vi "Autonomous.vi"   [LabVIEW 2015]
doc: "This VI starts when autonomous period begins, and will automatically be terminated when it ends. You can carry out timed or sensor driven operations directly to I/O or to subsystems without needing to return to the caller."
uses:
  <vilib>/Rock Robotics/Network Tables/NT Read String.vi
  <vilib>/Rock Robotics/Network Tables/NT Read Number.vi
  Framework/Robot Global Data.vi
  AutoTask/Implementation/AutoTask Operations.ctl
  AutoTask/Implementation/AutoTask Setpoints.ctl
  NavX/navX Library v2/navX Library v2.lvlib
types:
  T1 = typedef "AutoTask Setpoints.ctl" = cluster{"Operation":T2, "Setpoint":dbl, "Duration":dbl, "Speed":dbl, "Angle":dbl, "VDeadband":dbl, "Deadband":dbl}
  T2 = typedef "AutoTask Operations.ctl" = enum16{"Reserve", "Read Current", "Immediate", "DriveDistance", "AutoShoot", "FaceForward", "AutoAlign", "AutoTurn", "DriveToLine", "DriveToIncline", "DriveTillFlat"}
  T3 = typedef "navX Library v2.lvlib/Z900_navX_DeviceTypeDef.ctl" = cluster{"Interface":cluster{"Protocol":T4, "Update Rate (4Hz-60Hz)":u8, "navX Open TypeDef":variant}, "Notify Packet":refnum<notifier>, "Loop VI Refnum":refnum<vi>, "Ready to Close Occurrence Refnum":refnum<k4>}
  T4 = typedef "navX Library v2.lvlib/Z900_navX_ProtocolTypeDef.ctl" = enum16{"SERIAL", "I2C", "SPI"}
  T5 = cluster{"Yaw":dbl, "Roll":dbl, "Pitch":dbl, "Heading":dbl, "Fused Heading":dbl}
  T6 = typedef "WPI_EncoderDevRef.ctl" = cluster{"DevStatus":errorcluster, "EncoderIndex":T7, "CounterIndex":T8, "DistancePerCount":dbl, "Decoding Type":T9}
  T7 = typedef "FPGA_EncoderIdx.ctl" = enum8{"Enc 0", "Enc 1", "Enc 2", "Enc 3", "Enc 4", "Enc 5", "Enc 6", "Enc 7", "Invalid"}
  T8 = typedef "FPGA_CounterCtrSystemIndex.ctl" = enum8{"Ctr 0", "Ctr 1", "Ctr 2", "Ctr 3", "Ctr 4", "Ctr 5", "Ctr 6", "Ctr 7", "Invalid"}
  T9 = typedef "WPI_EncoderType.ctl" = enum16{"1x", "2x", "4x"}
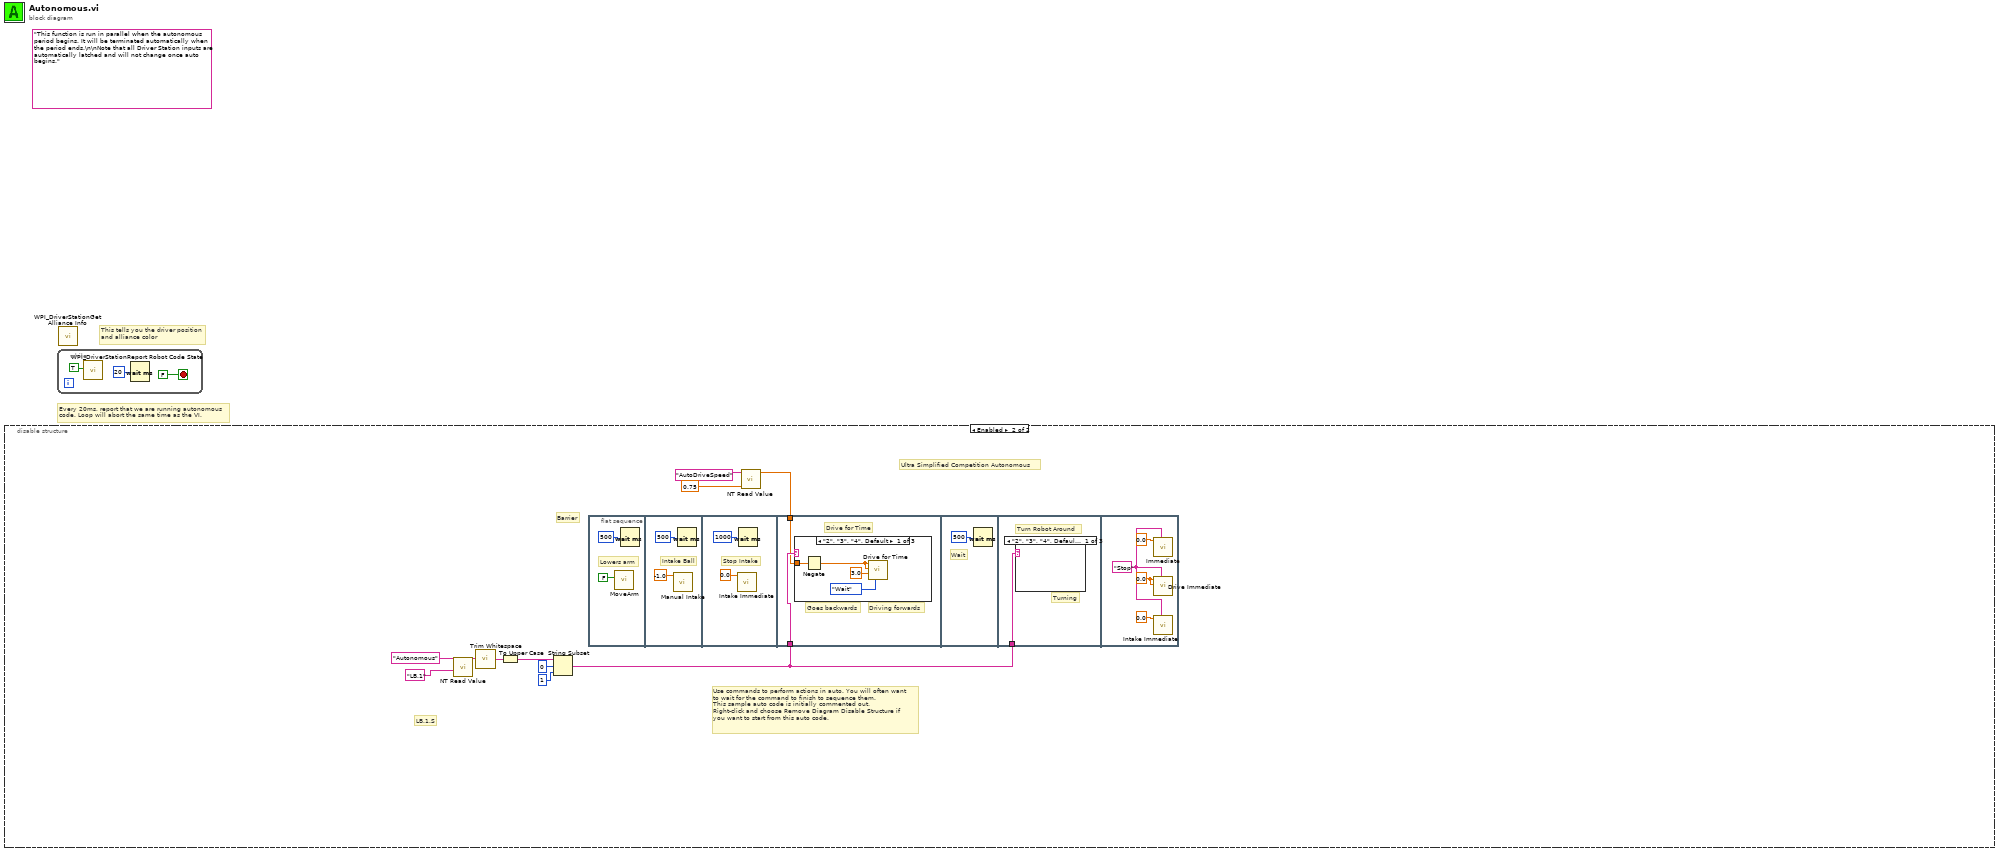
[diagram p0: block diagram]
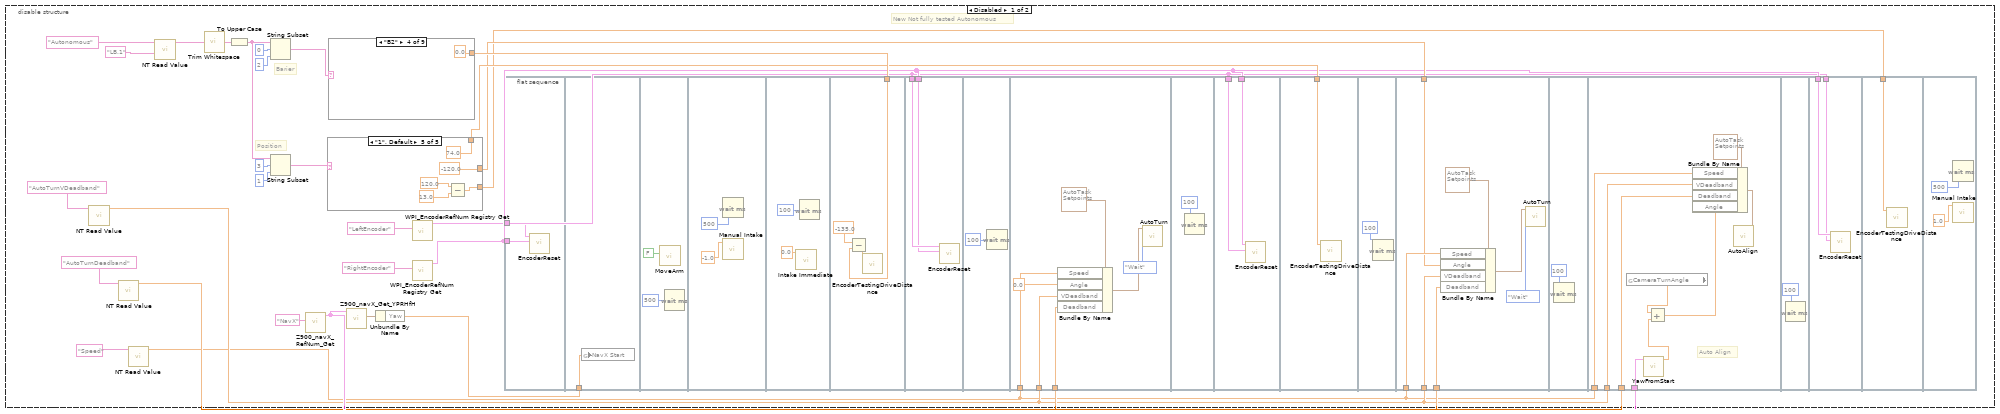
[diagram p2: hidden frame]
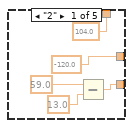
[diagram p3: hidden frame]
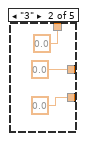
[diagram p4: hidden frame]
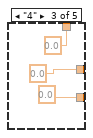
[diagram p5: hidden frame]
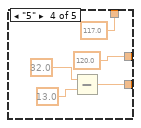
[diagram p6: hidden frame]
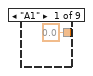
[diagram p7: hidden frame]
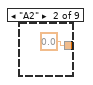
[diagram p8: hidden frame]
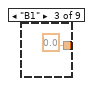
[diagram p9: hidden frame]
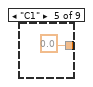
[diagram p10: hidden frame]
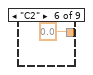
[diagram p11: hidden frame]
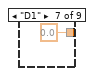
[diagram p12: hidden frame]
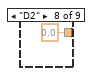
[diagram p13: hidden frame]
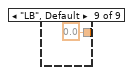
[diagram p14: hidden frame]
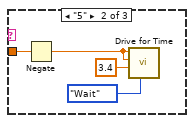
[diagram p15: hidden frame]
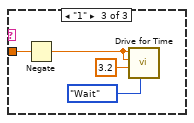
[diagram p16: hidden frame]
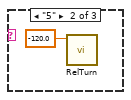
[diagram p17: hidden frame]
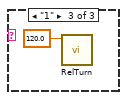
[diagram p18: hidden frame]
diagram:
  (unwired) "This function is run in parallel when the autonomous period begins. It will be terminated automatically when the period ends.\n\nNote that all Driver Station inputs are automatically latched and will not change once auto begins."
  # "Every 20ms, report that we are running autonomous\ncode. Loop will abort the same time as the VI."
  # "This tells you the driver position\nand alliance color"
  n1 = disable-structure shown="Enabled" {
    frame Disabled {
      # "New Not fully tested Autonomous"
      # "Barier"
      # "Position"
      n2 = call-poly <vilib>:"NT Read Value.vi"("Name"="AutoTurnVDeadband") -> ("Numeric"=w5:dbl)  [unwired: 9 in, 1 out]
      n3 = call-poly <vilib>:"NT Read Value.vi"("Name"="AutoTurnDeadband") -> ("Numeric"=w6:dbl)  [unwired: 9 in, 1 out]
      n4 = call-poly <vilib>:"NT Read Value.vi"("Name"="Speed") -> ("Numeric"=w4:dbl)  [unwired: 9 in, 1 out]
      n5 = call-poly <vilib>:"NT Read Value.vi"("Default Value"="LB.1", "Name"="Autonomous") -> ("String"=w23:string)  [unwired: 8 in, 1 out]
      n6 = call <vilib>:"Trim Whitespace.vi"("string"=w23) -> ("trimmed string"=w24:string)  [unwired: 1 in]
      n7 = To Upper Case(1:w24) -> (0:w21:string)
      n8 = String Subset(string=w21, offset (0)=0, length (rest)=2 ("length (rest)")) -> (substring=w20:string)
      n9 = String Subset(string=w21, offset (0)=3, length (rest)=1 ("length (rest)")) -> (substring=w10:string)
      n10 = call "Z900_navX_RefNum_Get.vi"("refnum name"="NavX") -> ("navX Device"=w7:T3)  [unwired: 9 in, 1 out]
      n11 = case shown="\"1\", Default" w10 {
        tunnel: [104.0 ("Distance") 0.0 ("Distance") 0.0 ("Distance") 117.0 ("Distance") 74.0 ("Distance")] -> w9
        tunnel: [-120.0 ("Distance") 0.0 ("Distance") 0.0 ("Distance") 120.0 ("Distance") -120.0 ("Distance")] -> w8
        tunnel: [w30 0.0 ("Distance") 0.0 ("Distance") w43 w48] -> w1
        frame "2" {
          n12 = Subtract(x=59.0 ("Distance"), y=13.0 ("Distance")) -> (x-y=w30:dbl)
        }
        frame "3" {
        }
        frame "4" {
        }
        frame "5" {
          n13 = Subtract(x=32.0 ("Distance"), y=13.0 ("Distance")) -> (x-y=w43:dbl)
        }
        frame "1", Default {
          n14 = Subtract(x=120.0 ("Distance"), y=13.0 ("Distance")) -> (x-y=w48:dbl)
        }
      }
      n15 = case shown="\"B2\"" w20 {
        tunnel: [0.0 ("Distance") 0.0 ("Distance") 0.0 ("Distance") 0.0 ("Distance") 0.0 ("Distance") 0.0 ("Distance") 0.0 ("Distance") 0.0 ("Distance") 0.0 ("Distance")] -> w14
        frame "A1" {
        }
        frame "A2" {
        }
        frame "B1" {
        }
        frame "B2" {
        }
        frame "C1" {
        }
        frame "C2" {
        }
        frame "D1" {
        }
        frame "D2" {
        }
        frame "LB", Default {
        }
      }
      n16 = call "Z900_navX_Get_YPRHfH.vi"("navX Device"=w7) -> ("YRPHfH"=w17:T5)  [unwired: 7 in, 3 out]
      n17 = Unbundle By Name(w17) -> ("Yaw"=w15:dbl)
      n18 = call <vilib>:"WPI_EncoderRefNum Registry Get.vi"("refnum name"="LeftEncoder") -> ("EncoderDevRef"=w2:T6)  [unwired: 9 in, 1 out]
      n19 = call <vilib>:"WPI_EncoderRefNum Registry Get.vi"("refnum name"="RightEncoder") -> ("EncoderDevRef"=w3:T6)  [unwired: 9 in, 1 out]
      n20 = flat-sequence {
        tunnel: w3 -> [w52]
        tunnel: w2 -> [w51]
        tunnel: w15 -> [w53]
        tunnel: w14 -> [w60]
        tunnel: w2 -> [w64]
        tunnel: w3 -> [w63]
        tunnel: w6 -> [w69]
        tunnel: w5 -> [w68]
        tunnel: w4 -> [w67]
        tunnel: w3 -> [w75]
        tunnel: w2 -> [w74]
        tunnel: w9 -> [w76]
        tunnel: w4 -> [w81]
        tunnel: w5 -> [w80]
        tunnel: w6 -> [w79]
        tunnel: w8 -> [w78]
        tunnel: w7 -> [w89]
        tunnel: w6 -> [w88]
        tunnel: w5 -> [w87]
        tunnel: w4 -> [w86]
        tunnel: w3 -> [w97]
        tunnel: w2 -> [w96]
        tunnel: w1 -> [w98]
        frame #0 {
          n21 = call "EncoderReset.vi"("EncoderDevRef 2"=w52, "EncoderDevRef"=w51) -> ()  [unwired: 10 in]
        }
        frame #1 {
          n22 = global write "Robot Global Data.vi" "NavX Start"(w53) -> ()
        }
        frame #2 {
          n23 = call "MoveArm.vi"("OnOff"=FALSE) -> ()  [unwired: 10 in, 1 out]
          n24 = Wait (ms)(milliseconds to wait=u32 500) -> ()  [unwired: 1 out]
        }
        frame #3 {
          n25 = Wait (ms)(milliseconds to wait=u32 500) -> ()  [unwired: 1 out]
          n26 = call "Manual Intake.vi"("Setpoint"=-1.0) -> ()  [unwired: 10 in, 1 out]
        }
        frame #4 {
          n27 = call "Intake Immediate.vi"("Setpoint"=0.0) -> ()  [unwired: 10 in, 1 out]
          n28 = Wait (ms)(milliseconds to wait=u32 100) -> ()  [unwired: 1 out]
        }
        frame #5 {
          n29 = Subtract(x=-135.0 ("Distance"), y=w60) -> (x-y=w61:dbl)
          n30 = call "EncoderTestingDriveDistance.vi"("Distance"=w61) -> ()  [unwired: 11 in]
        }
        frame #6 {
          n31 = call "EncoderReset.vi"("EncoderDevRef 2"=w63, "EncoderDevRef"=w64) -> ()  [unwired: 10 in]
        }
        frame #7 {
          n32 = Wait (ms)(milliseconds to wait=u32 100) -> ()  [unwired: 1 out]
        }
        frame #8 {
          n33 = Bundle By Name(cluster=T1 {"Operation"=enum."Reserve", "Setpoint"=0.0, "Duration"=0.0, "Speed"=0.0, "Angle"=0.0, "VDeadband"=0.0, "Deadband"=0.0} ("SubSystem Data"), "Speed"=w67, "Angle"=0.0, "VDeadband"=w68, "Deadband"=w69) -> (w70:T1)
          n34 = call "AutoTurn.vi"("Synchronization"=enum16{"Start", "Wait"}."Wait", "SubSystem Data"=w70) -> ()  [unwired: 8 in, 1 out]
        }
        frame #9 {
          n35 = Wait (ms)(milliseconds to wait=u32 100) -> ()  [unwired: 1 out]
        }
        frame #10 {
          n36 = call "EncoderReset.vi"("EncoderDevRef 2"=w74, "EncoderDevRef"=w75) -> ()  [unwired: 10 in]
        }
        frame #11 {
          n37 = call "EncoderTestingDriveDistance.vi"("Distance"=w76) -> ()  [unwired: 11 in]
        }
        frame #12 {
          n38 = Wait (ms)(milliseconds to wait=u32 100) -> ()  [unwired: 1 out]
        }
        frame #13 {
          n39 = Bundle By Name(cluster=T1 {"Operation"=enum."Reserve", "Setpoint"=0.0, "Duration"=0.0, "Speed"=0.0, "Angle"=0.0, "VDeadband"=0.0, "Deadband"=0.0} ("SubSystem Data"), "Speed"=w81, "Angle"=w78, "VDeadband"=w80, "Deadband"=w79) -> (w82:T1)
          n40 = call "AutoTurn.vi"("Synchronization"=enum16{"Start", "Wait"}."Wait", "SubSystem Data"=w82) -> ()  [unwired: 8 in, 1 out]
        }
        frame #14 {
          n41 = Wait (ms)(milliseconds to wait=u32 100) -> ()  [unwired: 1 out]
        }
        frame #15 {
          # "Auto Align"
          n42 = global read "Robot Global Data.vi" "CameraTurnAngle"() -> (w92:dbl)
          n43 = call "YawFromStart.vi"("navX Device"=w89) -> ("Yaw"=w93:dbl)  [unwired: 10 in]
          n44 = Add(x=w92, y=w93) -> (x+y=w94:dbl)
          n45 = Bundle By Name(cluster=T1 {"Operation"=enum."AutoAlign", "Setpoint"=0.0, "Duration"=0.0, "Speed"=0.0, "Angle"=0.0, "VDeadband"=0.0, "Deadband"=0.0} ("SubSystem Data"), "Speed"=w86, "VDeadband"=w87, "Deadband"=w88, "Angle"=w94) -> (w90:T1)
          n46 = call "AutoAlign.vi"("SubSystem Data"=w90) -> ()  [unwired: 10 in, 1 out]
        }
        frame #16 {
          n47 = Wait (ms)(milliseconds to wait=u32 100) -> ()  [unwired: 1 out]
        }
        frame #17 {
          n48 = call "EncoderReset.vi"("EncoderDevRef 2"=w96, "EncoderDevRef"=w97) -> ()  [unwired: 10 in]
        }
        frame #18 {
          n49 = call "EncoderTestingDriveDistance.vi"("Distance"=w98) -> ()  [unwired: 11 in]
        }
        frame #19 {
          n50 = Wait (ms)(milliseconds to wait=u32 500) -> ()  [unwired: 1 out]
          n51 = call "Manual Intake.vi"("Setpoint"=1.0) -> ()  [unwired: 10 in, 1 out]
        }
      }
    }
    frame Enabled {
      # "Ultra Simplified Competition Autonomous"
      # "LB.1.S"
      # "Barrier"
      # "Use commands to perform actions in auto. You will often want\nto wait for the command to finish to sequence them.\nThis sample auto code is initially commented out. \nRight-click and choose Remove Diagram Disable Structure if\nyou want to start from this auto code."
      n52 = call-poly <vilib>:"NT Read Value.vi"("Default Value"="LB.1", "Name"="Autonomous") -> ("String"=w112:string)  [unwired: 8 in, 1 out]
      n53 = call <vilib>:"Trim Whitespace.vi"("string"=w112) -> ("trimmed string"=w113:string)  [unwired: 1 in]
      n54 = To Upper Case(1:w113) -> (0:w114:string)
      n55 = String Subset(string=w114, offset (0)=0, length (rest)=1 ("length (rest)")) -> (substring=w116:string)
      n56 = flat-sequence {
        tunnel: w116 -> [w128]
        tunnel: w119 -> [w127]
        tunnel: w116 -> [w142]
        frame #0 {
          # "Lowers arm"
          n57 = call "MoveArm.vi"("OnOff"=FALSE) -> ()  [unwired: 10 in, 1 out]
          n58 = Wait (ms)(milliseconds to wait=u32 500) -> ()  [unwired: 1 out]
        }
        frame #1 {
          # "Intake Ball"
          n59 = call "Manual Intake.vi"("Setpoint"=-1.0) -> ()  [unwired: 10 in, 1 out]
          n60 = Wait (ms)(milliseconds to wait=u32 500) -> ()  [unwired: 1 out]
        }
        frame #2 {
          # "Stop Intake"
          n61 = call "Intake Immediate.vi"("Setpoint"=0.0) -> ()  [unwired: 10 in, 1 out]
          n62 = Wait (ms)(milliseconds to wait=u32 1000) -> ()  [unwired: 1 out]
        }
        frame #3 {
          # "Drive for Time"
          # "Goes backwards"
          # "Driving forwards"
          n63 = case shown="\"2\", \"3\", \"4\", Default" w128 {
            tunnel: w127 -> [w129 w133 w137]
            frame "2", "3", "4", Default {
              n64 = Negate(x=w129) -> (-x=w130:dbl)
              n65 = call "Drive for Time.vi"("Synchronization"=enum16{"Start", "Wait"}."Wait", "Seconds"=3.0, "Right Speed"=w130, "Left Speed"=w130) -> ()  [unwired: 6 in, 2 out]
            }
            frame "5" {
              n66 = Negate(x=w133) -> (-x=w134:dbl)
              n67 = call "Drive for Time.vi"("Synchronization"=enum16{"Start", "Wait"}."Wait", "Seconds"=3.4, "Right Speed"=w134, "Left Speed"=w134) -> ()  [unwired: 6 in, 2 out]
            }
            frame "1" {
              n68 = Negate(x=w137) -> (-x=w138:dbl)
              n69 = call "Drive for Time.vi"("Synchronization"=enum16{"Start", "Wait"}."Wait", "Seconds"=3.2, "Right Speed"=w138, "Left Speed"=w138) -> ()  [unwired: 6 in, 2 out]
            }
          }
        }
        frame #4 {
          # "Wait"
          n70 = Wait (ms)(milliseconds to wait=u32 500) -> ()  [unwired: 1 out]
        }
        frame #5 {
          # "Turn Robot Around"
          # "Turning"
          n71 = case shown="\"2\", \"3\", \"4\", Default" w142 {
            frame "2", "3", "4", Default {
            }
            frame "5" {
              n72 = call "RelTurn.vi"("Angle"=-120.0) -> ()  [unwired: 11 in]
            }
            frame "1" {
              n73 = call "RelTurn.vi"("Angle"=120.0) -> ()  [unwired: 11 in]
            }
          }
        }
        frame #6 {
          w145 = "Stop" ("Description")
          w148 = 0.0
          n74 = call "Immediate.vi"("Description"=w145, "Setpoint"=0.0) -> ()  [unwired: 9 in, 1 out]
          n75 = call "Drive Immediate.vi"("Description"=w145, "Right Setpoint"=w148, "Left Setpoint"=w148) -> ()  [unwired: 8 in, 1 out]
          n76 = call "Intake Immediate.vi"("Description"=w145, "Setpoint"=0.0) -> ()  [unwired: 9 in, 1 out]
        }
      }
      n77 = call-poly <vilib>:"NT Read Value.vi"("Default Value"=0.75, "Name"="AutoDriveSpeed") -> ("Numeric"=w119:dbl)  [unwired: 8 in, 1 out]
    }
  }
  n78 = while {
    stop <- FALSE stop-if-true
    n79 = call <vilib>:"WPI_DriverStationReport Robot Code State.vi"("Autonomous"=TRUE) -> ()  [unwired: 10 in, 1 out]
    n80 = Wait (ms)(milliseconds to wait=u32 20) -> ()  [unwired: 1 out]
  }
  n81 = call <vilib>:"WPI_DriverStationGet Alliance Info.vi"() -> ()  [unwired: 12 out]
